vi "Execute open-class-private-data-edit-time.vi"(6 "Mouse Position":T1, 8 "User VI Ref":refnum<vi>, 9 "Menu Item Tag Suffix":string, 10 "Remaining Items":refnum<vi>[](array[refnum]), 11 "Affected Items":T2) -> (0 "Fail transaction?":bool)   [LabVIEW 2022 SP3]
doc: "This VI is part of a plug-in for modifying the LabVIEW shortcut menus. This is the execute VI which is called when the shortcut menu is chosen by the user. It performs the action of the selected menu item."
uses:
  open-class-private-data-edit-time.ctl
  <vilib>/Utility/miscctls.llb/LVPositionTypeDef.ctl
panel:
  # "All controls on this panel except \"Affected Items\" have been locked to prevent accidental edits. Changing the control names or types, other than the elements of the \"Affected Items\" cluster will make the VI unusable as a menu plugin.\n\nSee Context Help for each control for details about its use."
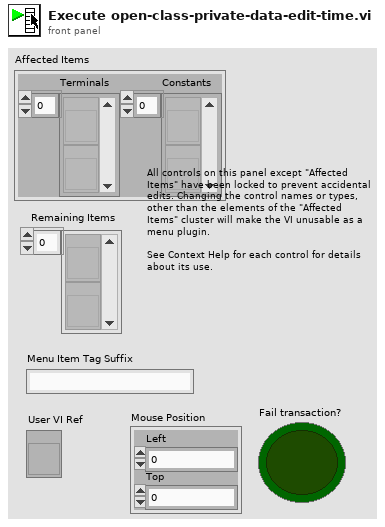
[diagram p1: front panel]
types:
  T1 = typedef "LVPositionTypeDef.ctl" = cluster{"Left":i32, "Top":i32}
  T2 = typedef "open-class-private-data-edit-time.ctl" = cluster{"Terminals":refnum<vi>[], "Constants":refnum<vi>[]}
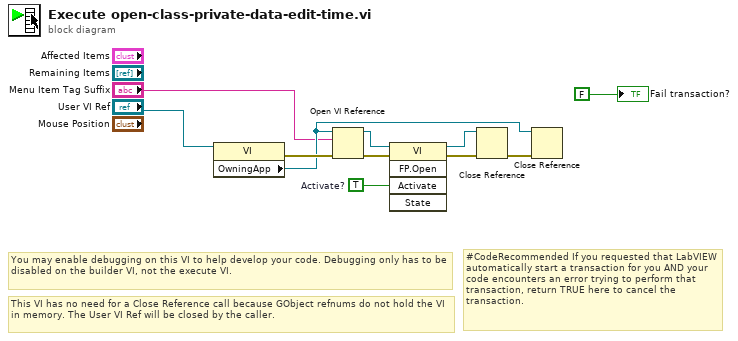
[diagram p0: block diagram]
diagram:
  w8 = TRUE  # Activate?
  # "You may enable debugging on this VI to help develop your code. Debugging only has to be disabled on the builder VI, not the execute VI."
  # "#CodeRecommended If you requested that LabVIEW automatically start a transaction for you AND your code encounters an error trying to perform that transaction, return TRUE here to cancel the transaction."
  # "This VI has no need for a Close Reference call because GObject refnums do not hold the VI in memory. The User VI Ref will be closed by the caller."
  n1 = property class="VI"(reference="User VI Ref") -> (error out=w10:errorcluster, "OwningApp"=w3:refnum<vi>)  [unwired: 1 in, 1 out]
  n2 = Open VI Reference(application reference (local)=w3, vi path="Menu Item Tag Suffix", error in (no error)=w10) -> (vi reference=w4:refnum<vi>, error out=w9:errorcluster)  [unwired: 3 in]
  n3 = invoke class="VI" method="FP.Open"(reference=w4, error in=w9, "Activate"=w8) -> (reference out=w6:refnum<vi>, error out=w7:errorcluster)  [unwired: 2 in, 3 out]
  n4 = Close Reference(reference=w6, error in (no error)=w7) -> (error out=w5:errorcluster)
  n5 = Close Reference(reference=w3, error in (no error)=w5) -> ()  [unwired: 1 out]
  "Fail transaction?" <- FALSE ("Fail transaction?")
